vi "Load_Data.vi"(2 "error in (no error)":errorcluster) -> (0 "error out":errorcluster, 1 "History Data":T1)   [LabVIEW 2021]
uses:
  <vilib>/Utility/file.llb/Read Delimited Spreadsheet (string).vi
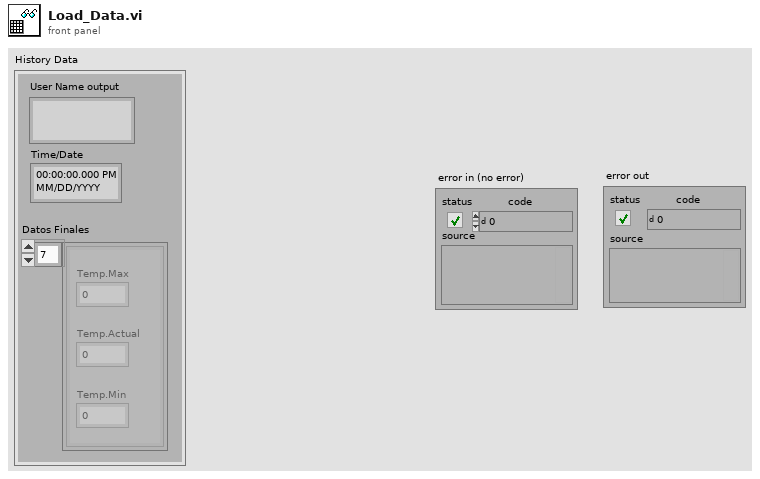
[diagram p1: front panel]
types:
  T1 = cluster{"User Name output":string, "Time/Date":timestamp, "Datos Finales":cluster{"Temp.Max":dbl, "Temp.Actual":dbl, "Temp.Min":dbl}[]}
  T2 = cluster{"String":string, timestamp, cluster{dbl, dbl, dbl}[]}
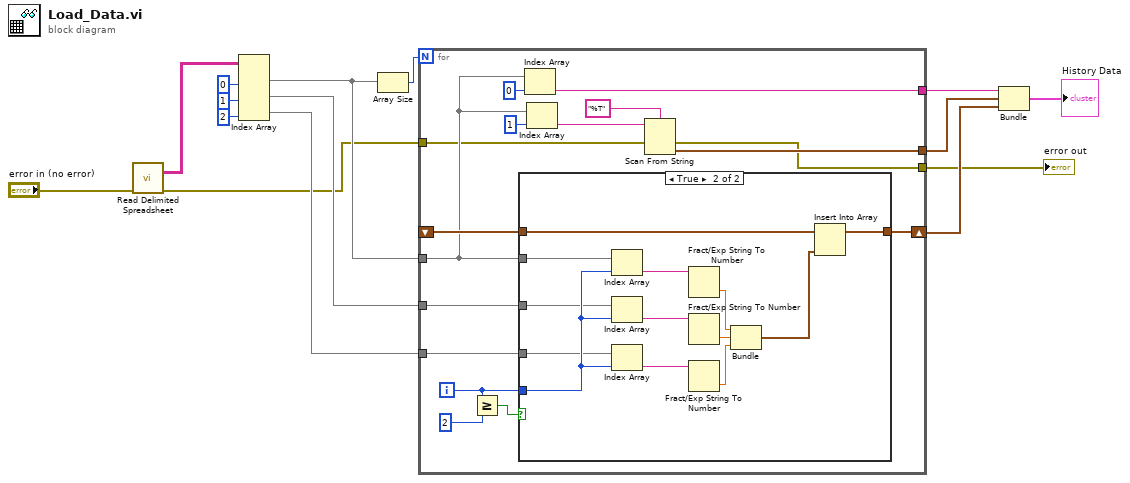
[diagram p0: block diagram]
diagram:
  n1 = call-poly <vilib>:"Read Delimited Spreadsheet.vi"("error in (no error)"="error in (no error)") -> ("all rows"=w15:string[][], "error out"=w3:errorcluster)  [unwired: 9 in, 4 out]
  n2 = Index Array(array=w15, index (col) #1=0 ("disabled index (col)"), index (col) #2=1 ("index (col)"), index (col) #3=2 ("index (col)")) -> (element #1=w7:string[], element #2=w10:string[], element #3=w9:string[])  [unwired: 3 in]
  n3 = Array Size(array=w7) -> (size(s)=w11:i32)
  n4 = for {
    N: w11 -> [_]
    tunnel: w7 -> [w19]
    tunnel: w10 -> [w28]
    tunnel: w9 -> [w27]
    shift-right: [w26] -> w8
    shift-left: _ -> [w25]
    tunnel: [w21] -> w2
    tunnel: [w18] -> w6
    tunnel: w3 -> [w17]
    tunnel: [w16] -> w1
    i -> [w29]
    n5 = Greater Or Equal?(x=w29, y=2) -> (x >= y?=w30:bool)
    n6 = case shown="True" w30 {
      tunnel: w29 -> [_ w45]
      tunnel: w19 -> [_ w44]
      tunnel: w28 -> [_ w43]
      tunnel: w27 -> [_ w42]
      tunnel: [w32 w35] -> w26
      tunnel: w25 -> [w32 w33]
      frame False {
      }
      frame True {
        n7 = Index Array(array=w44, index=w45) -> (element=w41:string)
        n8 = Index Array(array=w43, index=w45) -> (element=w39:string)
        n9 = Index Array(array=w42, index=w45) -> (element=w38:string)
        n10 = Fract/Exp String To Number(string=w41) -> (number=w40:dbl)  [unwired: 3 in, 1 out]
        n11 = Fract/Exp String To Number(string=w39) -> (number=w36:dbl)  [unwired: 3 in, 1 out]
        n12 = Fract/Exp String To Number(string=w38) -> (number=w37:dbl)  [unwired: 3 in, 1 out]
        n13 = Bundle(w40, w36, w37) -> (w34:cluster{dbl, dbl, dbl})  [unwired: 1 in]
        n14 = Insert Into Array(array=w33, new element=w34) -> (w35:cluster{dbl, dbl, dbl}[])  [unwired: 1 in]
      }
    }
    n15 = Index Array(array=w19, index=0) -> (element=w18:string)
    n16 = Index Array(array=w19, index=1) -> (element=w22:string)
    n17 = Scan From String(format string="%T", input string=w22, error in=w17) -> (error out=w16:errorcluster, output 1=w21:timestamp)  [unwired: 2 in, 2 out]
  }
  "error out" <- w1
  n18 = Bundle("String"=w6, w2, w8) -> (→"History Data":T2)  [unwired: 1 in]
